vi "Servo Main Loop.vi"(8 "error in (no error)":errorcluster, 9 "servo queue":refnum<queue>, 10 "servo notifier":refnum<notifier>, 11 "error queue":refnum<queue>) -> (0 "error out":errorcluster)   [LabVIEW 2020]
uses:
  GUI/Main GUI Loop/Handler.ctl
  Hardware/Actuators/Servos/Servo.lvclass
  C:/Users/jharw/Documents/1 Folder to Rule them All/UMD/Inflation-Apparatus/src/Hardware/General Hardware.lvclass
  Hardware/General Hardware.lvclass/General Hardware.ctl
  Hardware/Actuators/Servos/Servo.lvclass/Servo.ctl
  Hardware/General Hardware.lvclass
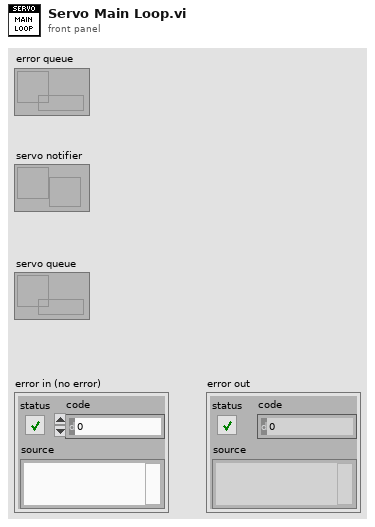
[diagram p1: front panel]
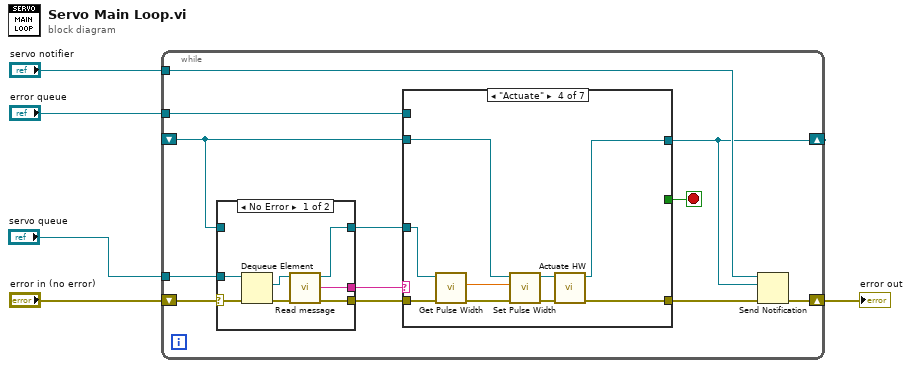
[diagram p0: block diagram]
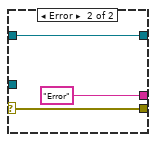
[diagram p2: hidden frame]
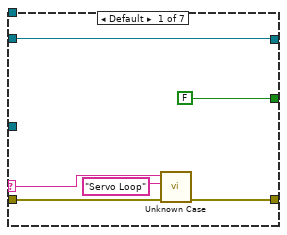
[diagram p3: hidden frame]
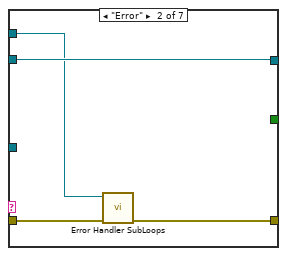
[diagram p4: hidden frame]
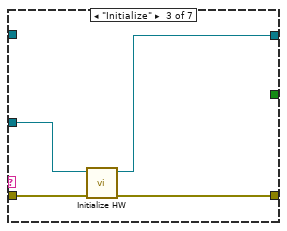
[diagram p5: hidden frame]
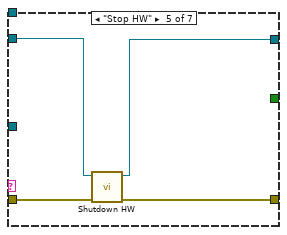
[diagram p6: hidden frame]
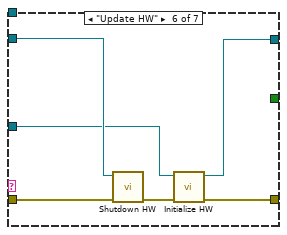
[diagram p7: hidden frame]
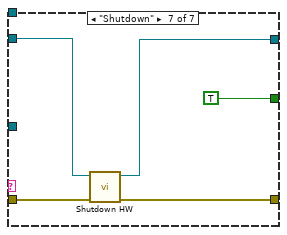
[diagram p8: hidden frame]
diagram:
  n1 = while {
    tunnel: "error queue" -> [w14]
    shift-right: [w8] -> w5
    shift-left: "error in (no error)" -> [w15]
    shift-right: [w6] -> _
    shift-left: _ -> [w12]
    tunnel: "servo queue" -> [w10]
    tunnel: "servo notifier" -> [w7]
    stop <- w11 stop-if-true
    n2 = case shown="No Error" w15 {
      selector: w15 -> [w18 w27]
      tunnel: [w24 w27] -> w17
      tunnel: [w22 "Error" ("message")] -> w16
      tunnel: [w23 w25] -> w13
      tunnel: w12 -> [_ w25]
      tunnel: w10 -> [w19 _]
      frame No Error {
        n3 = Dequeue Element(queue=w19, error in (no error)=w18) -> (element=w21:refnum<class "Servo.lvclass">, error out=w20:errorcluster)  [unwired: 1 in, 2 out]
        n4 = call "Read message.vi"("error in (no error)"=w20, "General Hardware in"=w21) -> ("error out"=w24:errorcluster, "message"=w22:string, "General Hardware out"=w23:refnum<class "Servo.lvclass">)  [unwired: 7 in]
      }
      frame Error {
      }
    }
    n5 = case shown="\"Actuate\"" w16 {
      selector: w16 -> [w31 _ _ _ _ _ _]
      tunnel: w17 -> [w33 w36 w41 w48 w54 w60 w64]
      tunnel: [w32 w35 w40 w49 w53 w58 w63] -> w9
      tunnel: w14 -> [_ w34 _ _ _ _ _]
      tunnel: w13 -> [_ _ w38 w47 _ w56 _]
      tunnel: [w29 w37 w39 w50 w51 w55 w61] -> w6
      tunnel: w12 -> [w29 w37 _ w43 w52 w57 w62]
      tunnel: [FALSE _ _ _ _ _ TRUE] -> w11
      frame Default {
        n6 = call "Unknown Case.vi"("error in (no error)"=w33, "source"="Servo Loop", "case"=w31) -> ("error out"=w32:errorcluster)  [unwired: 8 in]
      }
      frame "Error" {
        n7 = call "Error Handler SubLoops.vi"("error in"=w36, "main gui queue"=w34) -> ("error out"=w35:errorcluster)  [unwired: 9 in]
      }
      frame "Initialize" {
        n8 = call-dynamic "Initialize HW.vi"("error in (no error)"=w41, "Servo in"=w38) -> ("error out"=w40:errorcluster, "Servo out"=w39:refnum<class "Servo.lvclass">)  [unwired: 8 in]
      }
      frame "Actuate" {
        n9 = call "Get Pulse Width.vi"("error in (no error)"=w48, "Servo in"=w47) -> ("error out"=w46:errorcluster, "pulse width (micro-sec)"=w44:dbl)  [unwired: 7 in, 1 out]
        n10 = call "Set Pulse Width.vi"("error in (no error)"=w46, "pulse width (micro-sec)"=w44, "Servo in"=w43) -> ("error out"=w45:errorcluster, "Servo out"=w42:refnum<class "Servo.lvclass">)  [unwired: 7 in]
        n11 = call-dynamic "Actuate HW.vi"("error in (no error)"=w45, "Servo in"=w42) -> ("error out"=w49:errorcluster, "Servo out"=w50:refnum<class "Servo.lvclass">)  [unwired: 8 in]
      }
      frame "Stop HW" {
        n12 = call-dynamic "Shutdown HW.vi"("error in (no error)"=w54, "Servo in"=w52) -> ("error out"=w53:errorcluster, "Servo out"=w51:refnum<class "Servo.lvclass">)  [unwired: 8 in]
      }
      frame "Update HW" {
        n13 = call-dynamic "Shutdown HW.vi"("error in (no error)"=w60, "Servo in"=w57) -> ("error out"=w59:errorcluster)  [unwired: 8 in, 1 out]
        n14 = call-dynamic "Initialize HW.vi"("error in (no error)"=w59, "Servo in"=w56) -> ("error out"=w58:errorcluster, "Servo out"=w55:refnum<class "Servo.lvclass">)  [unwired: 8 in]
      }
      frame "Shutdown" {
        n15 = call-dynamic "Shutdown HW.vi"("error in (no error)"=w64, "Servo in"=w62) -> ("error out"=w63:errorcluster, "Servo out"=w61:refnum<class "Servo.lvclass">)  [unwired: 8 in]
      }
    }
    n16 = Send Notification(notification=w6, notifier=w7, error in (no error)=w9) -> (error out=w8:errorcluster)  [unwired: 1 out]
  }
  "error out" <- w5
